vi "PDSS - Write Comments to File.vi"(8 "error in":errorcluster, 10 "data":string, 11 "Base SCD Log File Folder (User must create)":path=path "C:/SCMP Logs") -> (0 "error out":errorcluster, 2 "Last Log Entry":string="\r", 3 "Entire Log File":string="\n", 5 "Today's SCD Log File":path)   [LabVIEW 2014]
doc: "This vi create or open file, which is save in format YYYYMMDD.txt. In this file are logs from CoMP-S Main program."
panel:
  out "date/time string":string="20141030"
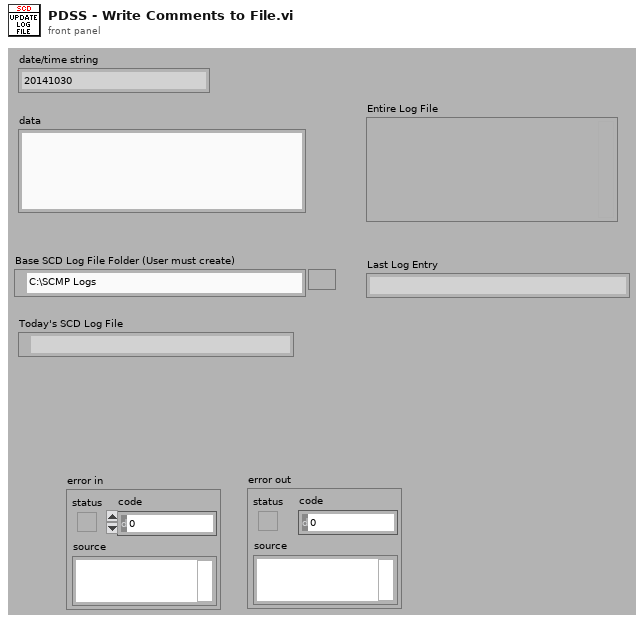
[diagram p1: front panel]
types:
  T1 = enum16{"open", "replace", "create", "open or create", "replace or create", "replace or create with confirmation"}
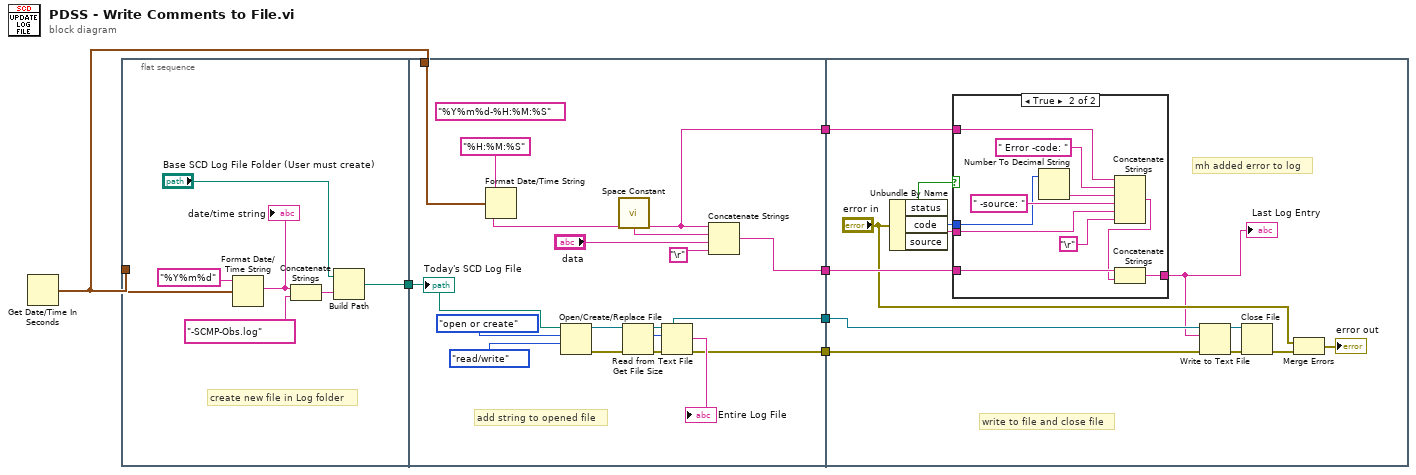
[diagram p0: block diagram]
diagram:
  n1 = Get Date/Time In Seconds() -> (seconds since 1Jan1904=w3:timestamp)
  n2 = flat-sequence {
    tunnel: w3 -> [w11]
    tunnel: [w7] -> w2
    tunnel: w3 -> [w21]
    tunnel: [w19] -> w6
    tunnel: [w20] -> w5
    tunnel: [w18] -> w4
    tunnel: w2 -> [w16]
    tunnel: [w14] -> w1
    tunnel: w6 -> [w38]
    tunnel: w5 -> [w42]
    tunnel: w4 -> [w37]
    tunnel: w1 -> [w36]
    frame #0 {
      # "create new file in Log folder"
      n3 = Format Date/Time String(time format string (%c)="%Y%m%d", seconds (now)=w11) -> (date/time string=w10:string)  [unwired: 1 in]
      "date/time string" <- w10
      n4 = Concatenate Strings(w10, "-SCMP-Obs.log" ("string")) -> (w9:string)
      n5 = Build Path(base path="Base SCD Log File Folder (User must create)", name or relative path=w9) -> (appended path=w7:path)
    }
    frame #1 {
      (unwired) "%Y%m%d-%H:%M:%S" ("time format string (%c)")
      # "add string to opened file"
      n6 = Format Date/Time String(time format string (%c)="%H:%M:%S", seconds (now)=w21) -> (date/time string=w18:string)  [unwired: 1 in]
      n7 = Open/Create/Replace File(file path (use dialog)=w16, operation (0:open)=T1."open or create", access (0:read/write)=enum16{"read/write", "read-only", "write-only"}."read/write") -> (refnum out=w28:refnum<file>, error out=w27:errorcluster)  [unwired: 1 in, 3 out]
      n8 = call <vilib>:"Space Constant.vi"() -> ("String"=w25:string)
      n9 = Get File Size(file=w28, error in=w27) -> (refnum out=w29:refnum<file>, size (in bytes)=w30:i64, 0:w15:errorcluster)
      n10 = Read from Text File(file (use dialog)=w29, count=w30, error in=w15) -> (refnum out=w20:refnum<file>, text=→"Entire Log File":string, error out=w14:errorcluster)  [unwired: 2 out]
      n11 = Concatenate Strings(w18, w25, "data", "\r") -> (w19:string)
      "Today's SCD Log File" <- w16
    }
    frame #2 {
      # "mh added error to log"
      # "write to file and close file"
      n12 = Unbundle By Name("error in") -> ("status"=w39:bool, "code"=w40:i32, "source"=w41:string)
      n13 = case shown="True" w39 {
        tunnel: w41 -> [_ w54]
        tunnel: w40 -> [_ w52]
        tunnel: w38 -> [w45 w49]
        tunnel: [w45 w48] -> w32
        tunnel: w37 -> [_ w47]
        frame False {
        }
        frame True {
          n14 = Number To Decimal String(number=w52) -> (decimal integer string=w51:string)  [unwired: 1 in]
          n15 = Concatenate Strings(w47, " Error -code: ", w51, " -source: ", w54, "\r") -> (w46:string)
          n16 = Concatenate Strings(w49, w46) -> (w48:string)
        }
      }
      "Last Log Entry" <- w32
      n17 = Write to Text File(file (use dialog)=w42, text=w32, error in=w36) -> (refnum out=w43:refnum<file>, error out=w44:errorcluster)  [unwired: 1 in, 1 out]
      n18 = Close File(refnum=w43, error in=w44) -> (error out=w34:errorcluster)  [unwired: 1 out]
      n19 = Merge Errors("error in", w34) -> (→"error out":errorcluster)
    }
  }
